vi "Receiver UI.vi"() -> ()   [LabVIEW 2021, in "Receiver.lvclass"]
uses:
  Receiver.lvclass
  Controls/Operation.ctl
  Controls/State Cluster.ctl
  FileExplorer2.0/Controls/Operations.ctl
  FileExplorer2.0/Controls/State.ctl
  Controls/User Event Operation.ctl
  Controls/Receiver Data Cluster.ctl
panel:
  out "Data":variant
  out "error out":errorcluster
  in  "error in (no error)":errorcluster
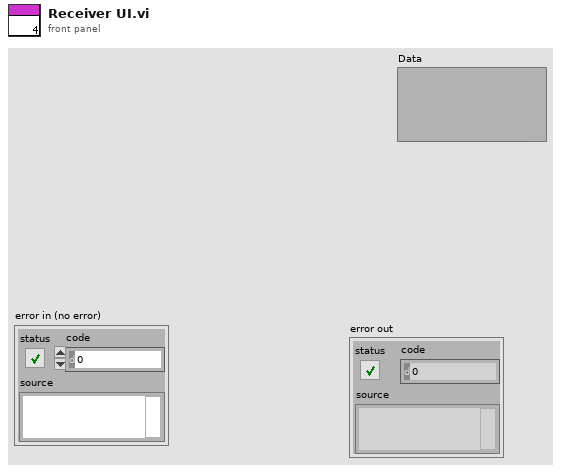
[diagram p1: front panel]
types:
  T1 = typedef "Receiver Data Cluster.ctl" = cluster{"Data":variant}
  T2 = typedef "User Event Operation.ctl" = enum16{"Obtain", "Generate", "Release"}
  T3 = typedef "State Cluster.ctl" = cluster{"State":string, "Data":variant}
  T4 = typedef "Operation.ctl" = enum16{"Create", "Enqueue", "Enqueue N", "Enstack", "Dequeue", "Flush", "Release"}
  T5 = typedef "State.ctl" = cluster{"State":string, "Data":variant}
  T6 = typedef "Operations.ctl" = enum16{"Create", "Enqueue", "Enqueue N", "Enstack", "Dequeue", "Flush", "Release"}
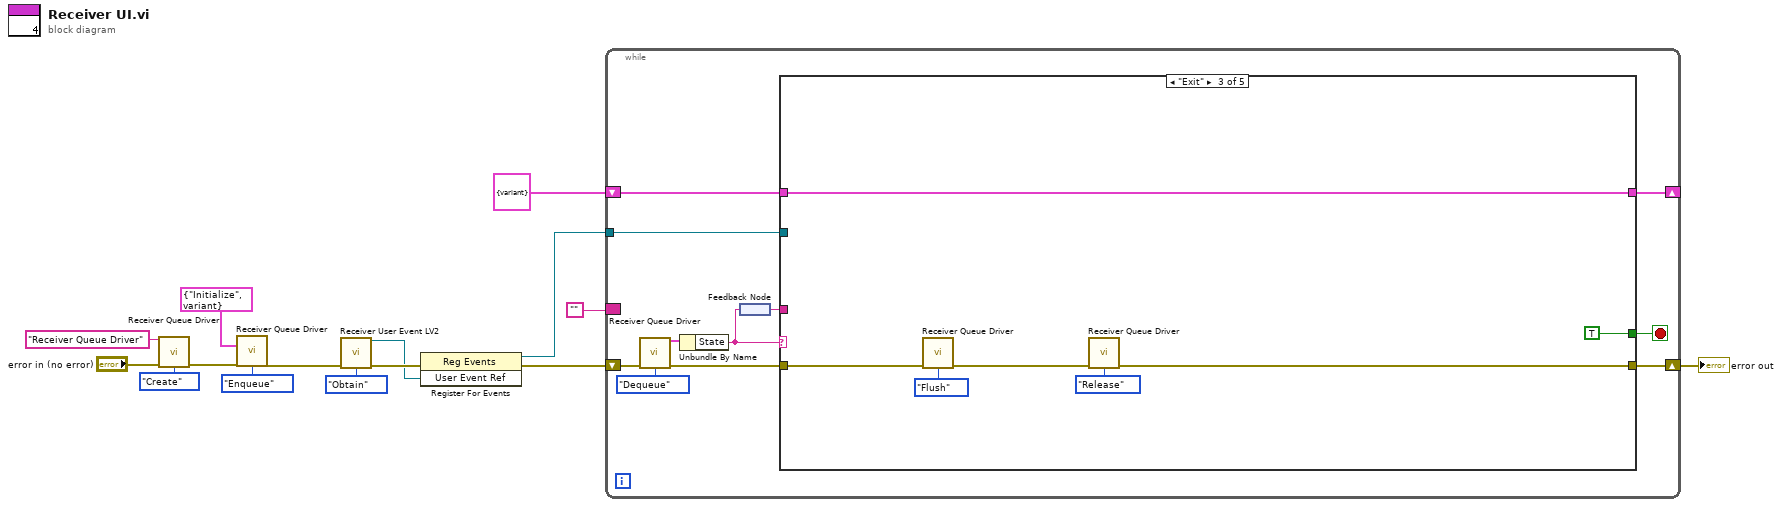
[diagram p0: block diagram]
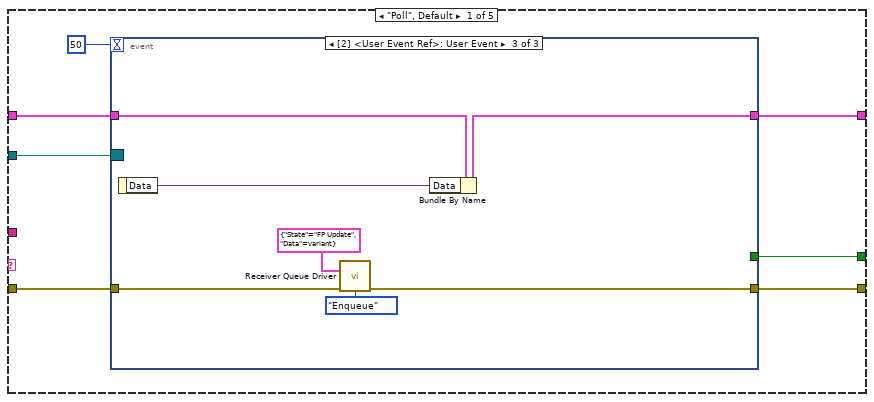
[diagram p2: hidden frame]
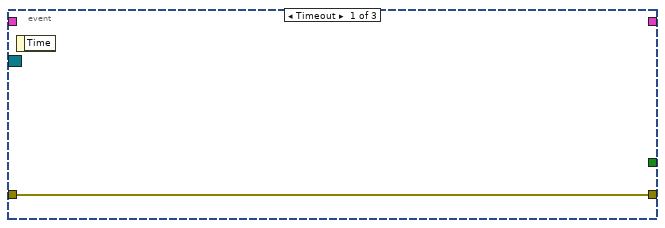
[diagram p3: hidden frame]
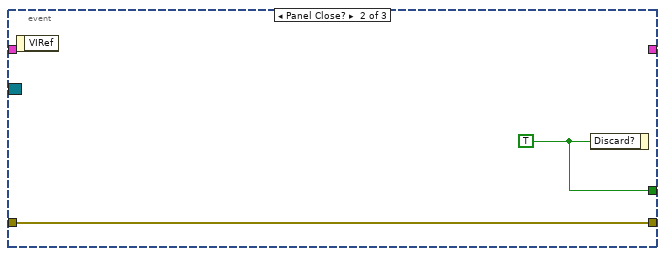
[diagram p4: hidden frame]
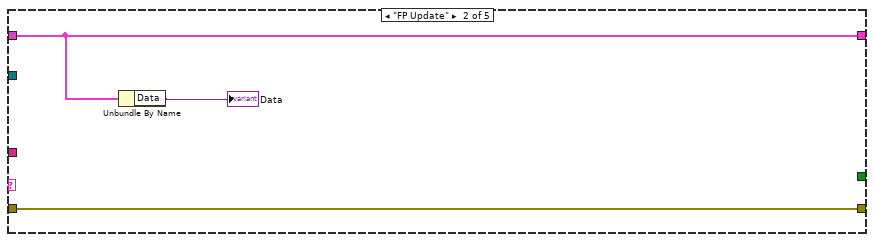
[diagram p5: hidden frame]
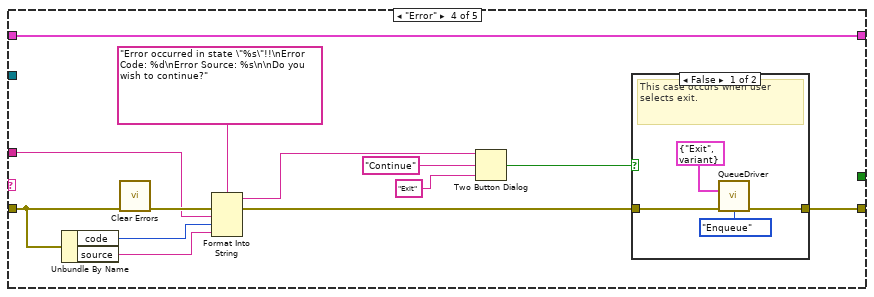
[diagram p6: hidden frame]
diagram:
  n1 = call "Receiver Queue Driver.vi"("Queue Name"="Receiver Queue Driver", "error in (no error)"="error in (no error)", "Operations"=Operation."Create") -> ("error out"=w14:errorcluster)  [unwired: 11 in, 1 out]
  n2 = call "Receiver Queue Driver.vi"("State"=T3 {"State"="Initialize", "Data"=variant}, "error in (no error)"=w14, "Operations"=Operation."Enqueue") -> ("error out"=w7:errorcluster)  [unwired: 11 in, 1 out]
  n3 = call "Receiver User Event LV2.vi"("Error In"=w7, "Operation"=User_Event_Operation."Obtain") -> ("User Event Ref"=w3:refnum<user-event>, "Error Out"=w6:errorcluster)  [unwired: 12 in]
  n4 = register-events(error in=w6, w3) -> (reference out=w2:refnum<event-registration>, error out=w4:errorcluster)  [unwired: 1 in]
  n5 = while {
    border: "" -> [_]
    shift-right: [w20] -> w8
    shift-left: w4 -> [w25]
    tunnel: w2 -> [w18]
    shift-right: [w16] -> _
    shift-left: T1 {"Data"=variant} -> [w17]
    stop <- w19 stop-if-true
    n6 = call "Receiver Queue Driver.vi"("error in (no error)"=w25, "Operations"=Operation."Dequeue") -> ("Dequeued Element"=w24:T3, "error out"=w23:errorcluster)  [unwired: 12 in]
    n7 = Unbundle By Name(w24) -> ("State"=w22:string)
    n8 = feedback-in #1(w22) -> ()
    n9 = feedback #1() -> (w21:string)
    n10 = case shown="\"Exit\"" w22 {
      tunnel: w23 -> [w33 w46 w53 w58 w73]
      tunnel: w21 -> [_ _ _ w55 _]
      tunnel: [w31 w46 w50 w59 w73] -> w20
      tunnel: [w30 _ TRUE ("Discard?") _ _] -> w19
      tunnel: w18 -> [w29 _ _ _ _]
      tunnel: w17 -> [w28 w44 w47 w54 w72]
      tunnel: [w27 w44 w47 w54 w72] -> w16
      frame "Poll", Default {
        n11 = event shown="[2] <User Event Ref>: User Event" {
          selector: w29 -> [_ _ _]
          dyn-events: _ -> [_ _ _]
          timeout: 50 -> [_ _ _]
          tunnel: w33 -> [w34 w36 w40]
          tunnel: [w34 w36 w39] -> w31
          tunnel: [_ w35 _] -> w30
          tunnel: w28 -> [_ _ w43]
          tunnel: [_ _ w41] -> w27
          event Timeout {
            n12 = event-data() -> ()  [unwired: 1 in, 1 out]
          }
          event Panel Close? {
            w35 = TRUE ("Discard?")
            n13 = event-data() -> ()  [unwired: 1 in, 1 out]
            n14 = event-data("Discard?"=w35) -> ()  [unwired: 1 in, 1 out]
          }
          event User Event {
            n15 = event-data() -> ("Data"=w42:variant)  [unwired: 1 in]
            n16 = call "Receiver Queue Driver.vi"("State"=T3 {"State"="FP Update", "Data"=variant}, "error in (no error)"=w40, "Operations"=Operation."Enqueue") -> ("error out"=w39:errorcluster)  [unwired: 11 in, 1 out]
            n17 = Bundle By Name(cluster=w43, "Data"=w42) -> (w41:T1)
          }
        }
      }
      frame "FP Update" {
        n18 = Unbundle By Name(w44) -> ("Data"=→"Data":variant)
      }
      frame "Exit" {
        n19 = call "Receiver Queue Driver.vi"("error in (no error)"=w53, "Operations"=Operation."Flush") -> ("error out"=w51:errorcluster)  [unwired: 12 in, 1 out]
        n20 = call "Receiver Queue Driver.vi"("error in (no error)"=w51, "Operations"=Operation."Release") -> ("error out"=w50:errorcluster)  [unwired: 12 in, 1 out]
      }
      frame "Error" {
        n21 = Unbundle By Name(w58) -> ("code"=w56:i32, "source"=w57:string)
        n22 = call <vilib>:"Clear Errors.vi"("error in (no error)"=w58) -> ("error out"=w66:errorcluster)  [unwired: 5 in, 1 out]
        n23 = Format Into String(format string="Error occurred in state \"%s\"!!\nError Code: %d\nError Source: %s\n\nDo you wish to continue?", error in=w66, w55, w56, w57) -> (resulting string=w64:string, error out=w61:errorcluster)  [unwired: 1 in]
        n24 = Two Button Dialog(message=w64, 1:"Exit" ("F button name (\"Cancel\")"), 2:"Continue" ("T button name (\"OK\")")) -> (T button?=w60:bool)
        n25 = case shown="False" w60 {
          tunnel: w61 -> [w70 w71]
          tunnel: [w69 w71] -> w59
          frame False {
            # "This case occurs when user selects exit."
            n26 = call "QueueDriver.vi"("State"=T5 {"State"="Exit", "Data"=variant}, "error in (no error)"=w70, "Operations"=Operations."Enqueue") -> ("error out"=w69:errorcluster)  [unwired: 11 in, 1 out]
          }
          frame True {
            # "This case occurs when user selects to continue."
          }
        }
      }
      frame "Initialize " {
      }
    }
  }
  "error out" <- w8
